vi "DCC_Initialize.vi"(6 "Use Specified DLL and INI Path":bool, 8 "Error In":errorcluster, 9 "Mode":u16(ring) items=["Hardware Mode", "Simulation Mode"], 11 "Init Cluster":T1) -> (0 "Error Out":errorcluster, 1 "Number of \nUsable Modules":i16, 2 "Module Array":i16[](array[numeric]), 3 "DLL path":path=path "C:/Program Files (x86)/BH/SPCM/DLL/spcm64.dll" caption="DLL Path", 4 "Array of\nUsable Modules":T2[](array[typedef]), 5 "Serial Number":string[](array[string]))   [LabVIEW 2019]
doc: "Establishes communication with the cards installed in the computer system or with an external device which includes DCC cards. \nIt also checks how many cards are available and ask the user which cards are going to be used. Further, it prepares the cards for further driver operations. \nTherefore, call this VI before calling other driver VIs for this device. Generally, you need to call the <b>Initialize</b> VI only once at the beginning of an application.\n\nOctober 2018\nFrank Quadt & Stefan Smietana\ninfo@becker-hickl.com"
uses:
  DCC_Controls/DCC_ModuleInfoCluster.ctl
  DCC_Controls/DCC_InitCluster.ctl
  DCC_Controls/DCC_ModuleTypes.ctl
panel:
  # "This function initialise the DCC modules specified by the user if they are not blocked by other applications.\nThe user will be asked which module he or she wants to use."
  # "(c) 2021 Becker & Hickl GmbH\n     All Rights Reserved."
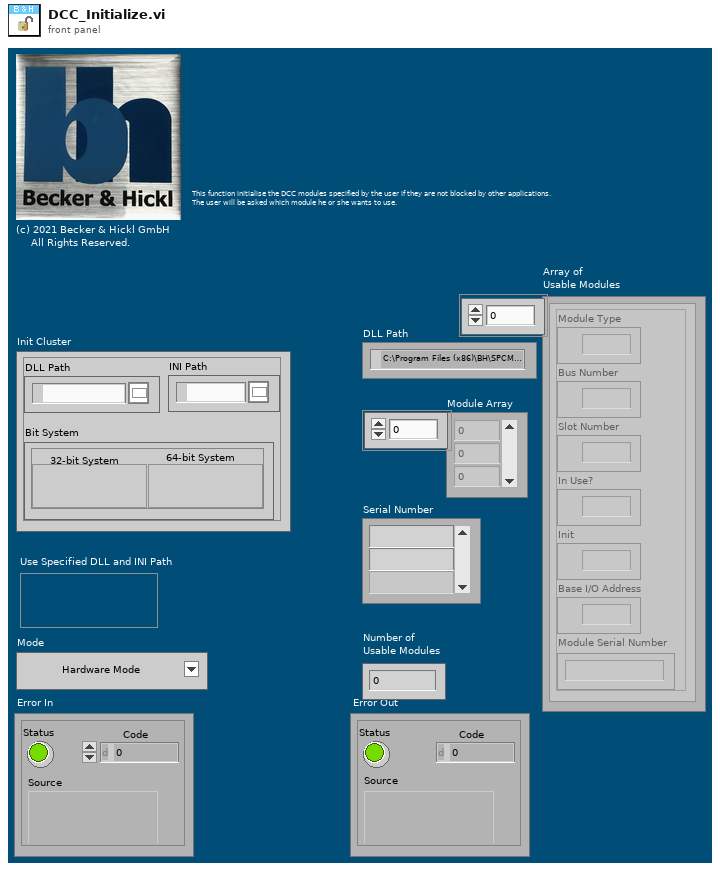
[diagram p1: front panel]
types:
  T1 = typedef "DCC_InitCluster.ctl" = cluster{"DLL Path":path, "INI Path":path, "Bit System":cluster{"32-bit System":bool, "64-bit System":bool}}
  T2 = typedef "DCC_ModuleInfoCluster.ctl" = cluster{"Module Type":i16, "Bus Number":i16, "Slot Number":i16, "In Use?":i16, "Init":i16, "Base I/O Address":u16, "Module Serial Number":string}
  T3 = typedef "DCC_ModuleTypes.ctl" = i16
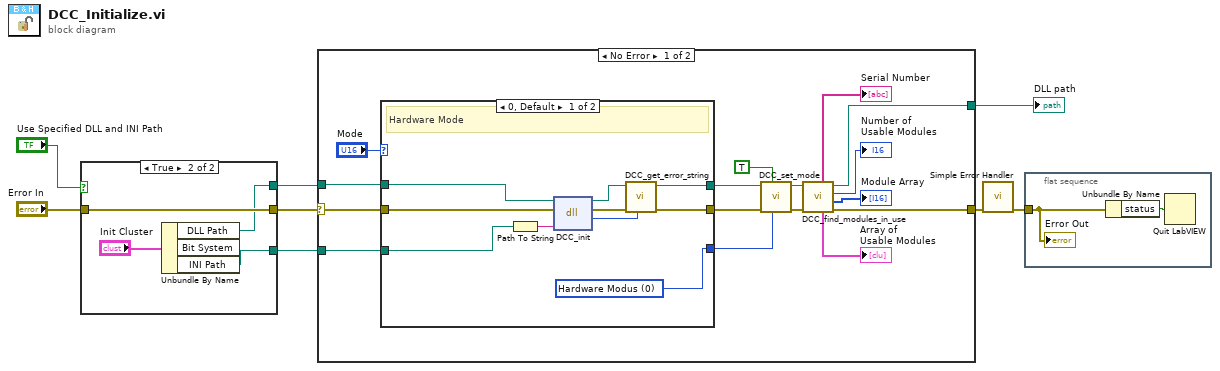
[diagram p0: block diagram]
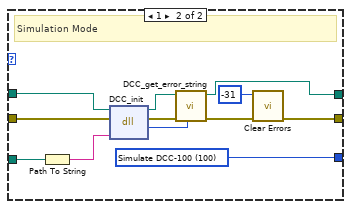
[diagram p2: hidden frame]
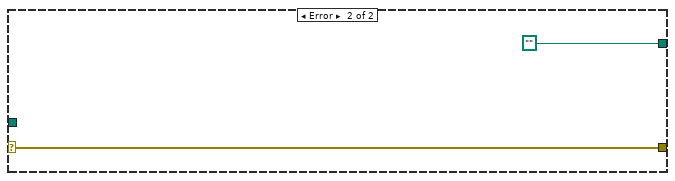
[diagram p3: hidden frame]
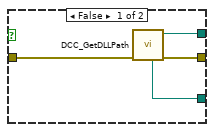
[diagram p4: hidden frame]
diagram:
  n1 = case shown="True" "Use Specified DLL and INI Path" {
    tunnel: [w12 w14] -> w8
    tunnel: [w9 w13] -> w2
    tunnel: [w11 w16] -> w1
    tunnel: "Error In" -> [w10 w16]
    frame False {
      n2 = call "DCC_GetDLLPath.vi"("Error In"=w10) -> ("Error Out"=w11:errorcluster, "DLL Path"=w12:path, "DCC Folder Path"=w9:path)  [unwired: 7 in, 1 out]
    }
    frame True {
      n3 = Unbundle By Name("Init Cluster") -> ("DLL Path"=w14:path, "INI Path"=w13:path)  [unwired: 1 out]
    }
  }
  n4 = case shown="No Error" w1 {
    selector: w1 -> [w30 w56]
    tunnel: w8 -> [w32 _]
    tunnel: w2 -> [w31 _]
    tunnel: [w27 path ""] -> w3
    tunnel: [w28 w56] -> w7
    frame No Error {
      n5 = case shown="0, Default" "Mode" {
        tunnel: w32 -> [w40 w47]
        tunnel: w31 -> [w33 w49]
        tunnel: [w42 w43] -> w18
        tunnel: [w41 w44] -> w20
        tunnel: w30 -> [w39 w46]
        tunnel: [w38 w45] -> w17
        frame 0, Default {
          w38 = T3 0 items=["Hardware Modus"=0, "Simulate DCC-100"=100, "Simulate DCU- 400/800"=200] ("Modul Type to Simulate")
          # "Hardware Mode"
          n6 = Path To String(path=w33) -> (string=w34:string)
          n7 = dll-call lib="C:/Program Files/BH/DCC/DLL/dcc32.dll" fn="DCC_init"(path in=w40, error in=w39, "Ini_file"=w34) -> (path out=w36:path, error out=w37:errorcluster, "return type"=w35:i16)  [unwired: 2 in]
          n8 = call "DCC_get_error_string.vi"("Error ID"=w35, "Error In"=w37, "DLL Path"=w36) -> ("Error Out"=w41:errorcluster, "DLL Path"=w42:path)  [unwired: 6 in, 1 out]
        }
        frame 1 {
          w45 = T3 100 items=["Hardware Modus"=0, "Simulate DCC-100"=100, "Simulate DCU- 400/800"=200] ("Modul Type to Simulate")
          # "Simulation Mode"
          n9 = Path To String(path=w49) -> (string=w48:string)
          n10 = dll-call lib="C:/Program Files/BH/DCC/DLL/dcc32.dll" fn="DCC_init"(path in=w47, error in=w46, "Ini_file"=w48) -> (path out=w53:path, error out=w52:errorcluster, "return type"=w50:i16)  [unwired: 2 in]
          n11 = call "DCC_get_error_string.vi"("Error ID"=w50, "Error In"=w52, "DLL Path"=w53) -> ("Error Out"=w51:errorcluster, "DLL Path"=w43:path)  [unwired: 6 in, 1 out]
          n12 = call <vilib>:"Clear Errors.vi"("error in (no error)"=w51, "specific error code to clear (0: all)"=-31) -> ("error out"=w44:errorcluster)  [unwired: 4 in, 1 out]
        }
      }
      n13 = call "DCC_set_mode.vi"("Modul Type to Simulate"=w17, "Force Use"=TRUE, "Error In"=w20, "DLL Path"=w18) -> ("Error Out"=w21:errorcluster, "DLL Path"=w19:path)  [unwired: 6 in]
      n14 = call "DCC_find_modules_in_use.vi"("Error In"=w21, "DLL Path"=w19) -> ("Error Out"=w28:errorcluster, "Module Array"=→"Module Array":i16[], "Number of \nUsable Modules"=→"Number of \nUsable Modules":i16, "DLL Path"=w27:path, "Array of\nUsable Modules"=→"Array of\nUsable Modules":T2[], "Module S/Ns"=→"Serial Number":string[])  [unwired: 4 in]
    }
    frame Error {
    }
  }
  "DLL path" <- w3
  n15 = call <vilib>:"Simple Error Handler.vi"("error in (no error)"=w7) -> ("error out"=w6:errorcluster)  [unwired: 4 in, 4 out]
  n16 = flat-sequence {
    tunnel: w6 -> [w58]
    frame #0 {
      n17 = Unbundle By Name(w58) -> ("status"=w57:bool)
      n18 = Quit LabVIEW(quit? (T)=w57) -> ()
      "Error Out" <- w58
    }
  }
